vi "Msg.vi"(7 "Actor in":refnum<class "Actor.lvclass">, 11 "Setup Msg in":refnum<class "Setup Msg.lvclass">) -> (5 "Actor out":refnum<class "Actor.lvclass">)   [LabVIEW 2021, in "jettl.lvlib" / "Setup Msg.lvlib" / "Setup Msg.lvclass"]
uses:
  Setup Msg.lvclass
  Temporary Actor/Actor/Actor.lvclass
  Setup/Setup.lvclass
  Setup Msg.lvclass/Setup Msg.ctl
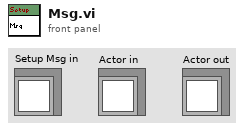
[diagram p1: front panel]
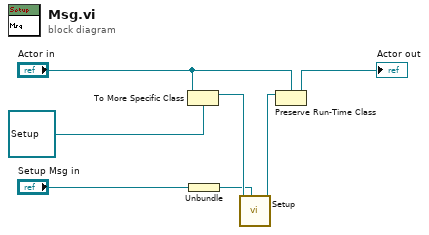
[diagram p0: block diagram]
diagram:
  n1 = To More Specific Class(target class=refnum<class "Setup.lvclass"> refnum ("Setup.lvlib:Setup.lvclass"), reference="Actor in") -> (specific class reference=w3:refnum<class "Setup.lvclass">)  [unwired: 1 in, 1 out]
  n2 = Unbundle "Unbundle"("Setup Msg in") -> (w1:refnum<class "Sender.lvclass">)
  n3 = call-dynamic "Setup.vi"("Sender"=w1, "Setup in"=w3) -> ("Setup out"=w2:refnum<class "Setup.lvclass">)  [unwired: 9 in]
  n4 = Preserve Run-Time Class(object in=w2, 2:"Actor in") -> (object out=→"Actor out":refnum<class "Actor.lvclass">)  [unwired: 1 in, 1 out]
